vi "CreateNewSystemDefinition.vi"(8 "error in (no error)":errorcluster, 10 "System Definition Name":string, 11 "VeriStandScriptingTestCase in":refnum<class "VeriStandScriptingTestCase.lvclass">) -> (0 "error out":errorcluster, 3 "VeriStandScriptingTestCase out":refnum<class "VeriStandScriptingTestCase.lvclass">)   [LabVIEW 2017, in "VeriStandScriptingTestCase.lvclass"]
uses:
  VeriStandScriptingTestCase.lvclass
  VeriStandTestUtilities/VeriStandTestUtilities.lvlib
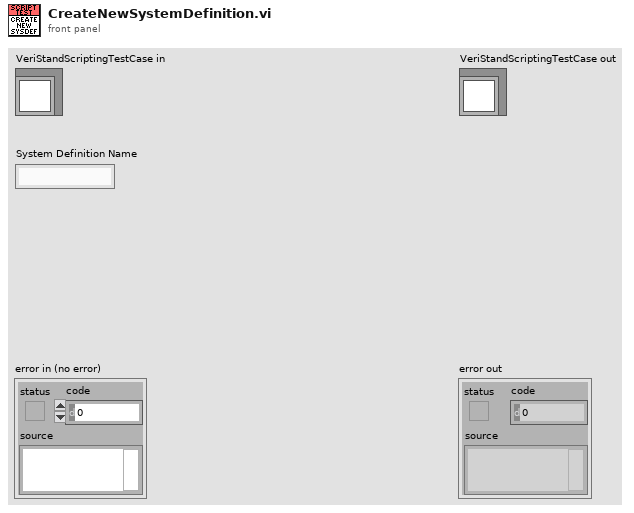
[diagram p1: front panel]
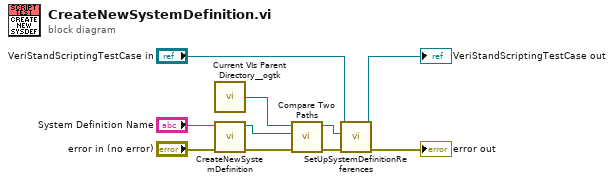
[diagram p0: block diagram]
diagram:
  n1 = call <userlib>:"Current VIs Parent Directory__ogtk.vi"() -> ("Parent Directory (+ Relative)"=w6:path)  [unwired: 5 in]
  n2 = call "CreateNewSystemDefinition.vi"("error in"="error in (no error)", "System Definition Name"="System Definition Name") -> ("error out"=w8:errorcluster, "System Definition Path"=w7:path)  [unwired: 8 in]
  n3 = call <vilib>:"Compare Two Paths.vi"("error in (no error)"=w8, "Path 2"=w7, "Path 1"=w6) -> ("error out"=w5:errorcluster, "Relative Path from 1 to 2"=w3:path)  [unwired: 5 in, 2 out]
  n4 = call "SetUpSystemDefinitionReferences.vi"("error in"=w5, "Relative Path to SysDef"=w3, "VeriStandScriptingTestCase in"="VeriStandScriptingTestCase in") -> ("error out"=→"error out":errorcluster, "VeriStandScriptingTestCase out"=→"VeriStandScriptingTestCase out":refnum<class "VeriStandScriptingTestCase.lvclass">)  [unwired: 7 in]
